vi "ChangeMode.vi"(8 "error in (no error)":errorcluster, 9 "Save to TblHist? (T)":bool=TRUE, 10 "ModeChange Cluster":T1, 11 "ModeCol in":refnum<class "ModeCol.lvclass">) -> (0 "error out":errorcluster, 3 "ModeCol out":refnum<class "ModeCol.lvclass">)   [LabVIEW 2013, in "ModeCol.lvclass"]
doc: "Update Mode cell to user-selected value. This VI can be \"programatically\" called to enforce allowed Modes inside loops without saving to the undo/redo history by setting \"Save to TblHist?\" to False."
uses:
  ModeCol.lvclass
  TypeDefs/ModeChange.ctl
  <vilib>/Utility/miscctls.llb/LVRowAndColumnTypeDef.ctl
  TypeDefs/TableHistory.ctl
  TypeDefs/TableArray.ctl
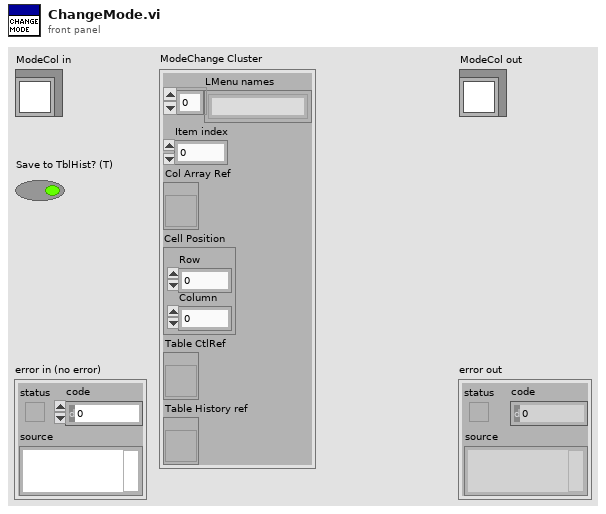
[diagram p1: front panel]
types:
  T1 = typedef "ModeChange.ctl" = cluster{"LMenu names":string[], "Item index":i32, "Col Array Ref":refnum<vi>, "Cell Position":T2, "Table CtlRef":refnum<vi>, "Table History ref":refnum<vi>}
  T2 = typedef "LVRowAndColumnTypeDef.ctl" = cluster{"Row":i32, "Column":i32}
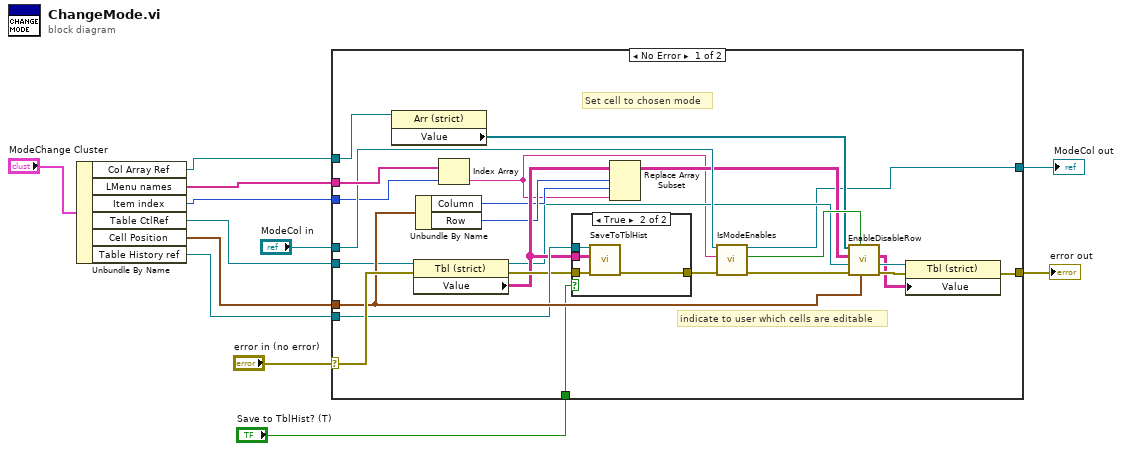
[diagram p0: block diagram]
diagram:
  n1 = Unbundle By Name("ModeChange Cluster") -> ("Col Array Ref"=w4:refnum<vi>, "LMenu names"=w2:string[], "Item index"=w3:i32, "Table CtlRef"=w7:refnum<vi>, "Cell Position"=w8:T2, "Table History ref"=w6:refnum<vi>)
  n2 = case shown="No Error" "error in (no error)" {
    selector: "error in (no error)" -> [w34 w44]
    tunnel: [w15 w44] -> w11
    tunnel: [w14 w43] -> w9
    tunnel: "ModeCol in" -> [w35 w43]
    tunnel: w2 -> [w37 _]
    tunnel: w4 -> [w36 _]
    tunnel: w7 -> [w31 _]
    tunnel: w8 -> [w32 _]
    tunnel: w6 -> [w30 _]
    tunnel: w3 -> [w33 _]
    tunnel: "Save to TblHist? (T)" -> [w13 _]
    frame No Error {
      # "Set cell to chosen mode"
      # "indicate to user which cells are editable"
      n3 = property class="Arr (strict)"(reference=w36) -> ("Value"=w26:refnum<class "Column.lvclass">[])  [unwired: 1 in, 2 out]
      n4 = property class="Tbl (strict)"(reference=w31, error in=w34) -> (reference out=w22:refnum<vi>, error out=w27:errorcluster, "Value"=w25:string[][])
      n5 = Unbundle By Name(w32) -> ("Column"=w23:i32, "Row"=w24:i32)
      n6 = Index Array(array=w37, index=w33) -> (element=w16:string)
      n7 = case shown="True" w13 {
        tunnel: w30 -> [_ w42]
        tunnel: w27 -> [w38 w41]
        tunnel: w25 -> [_ w40]
        tunnel: [w38 w39] -> w18
        frame False {
        }
        frame True {
          n8 = call "SaveToTblHist.vi"("error in (no error)"=w41, "OldTable (reset)"=w40, "Table History ref"=w42) -> ("error out"=w39:errorcluster)  [unwired: 8 in]
        }
      }
      n9 = Replace Array Subset(array=w25, new element=w16, index (row)=w24, index (col)=w23) -> (w21:string[][])
      n10 = call "IsModeEnables.vi"("error in (no error)"=w18, "Mode value"=w16, "ModeCol in"=w35) -> ("error out"=w29:errorcluster, "Disable / Enable"=w28:bool, "ModeCol out"=w14:refnum<class "ModeCol.lvclass">)  [unwired: 6 in]
      n11 = call "EnableDisableRow.vi"("Cell Position"=w32, "Disable / Enable"=w28, "error in (no error)"=w29, "Table CtlRef In"=w22, "Table Data in"=w21, "Col Array in"=w26) -> ("error out"=w19:errorcluster, "Table CtlRef Out"=w20:refnum<vi>, "Table Data out"=w17:string[][])  [unwired: 3 in]
      n12 = property class="Tbl (strict)"(reference=w20, error in=w19, "Value"=w17) -> (error out=w15:errorcluster)  [unwired: 1 out]
    }
    frame Error {
    }
  }
  "error out" <- w11
  "ModeCol out" <- w9
